vi "Home.vi"() -> ()   [LabVIEW 2015]
uses:
  <userlib>/QMH/Message Queue/Support/Enqueue Message (Single).vi
  <vilib>/Utility/error.llb/Error Cluster From Error Code.vi
  <vilib>/ErrorRing/Error Ring.xnode
  <userlib>/QMH/User Event - Stop/User Event - Stop.lvlib
  <userlib>/QMH/Message Queue/Message Queue.lvlib
panel:
  in  "Exit":bool
  in  "HostThread":variant
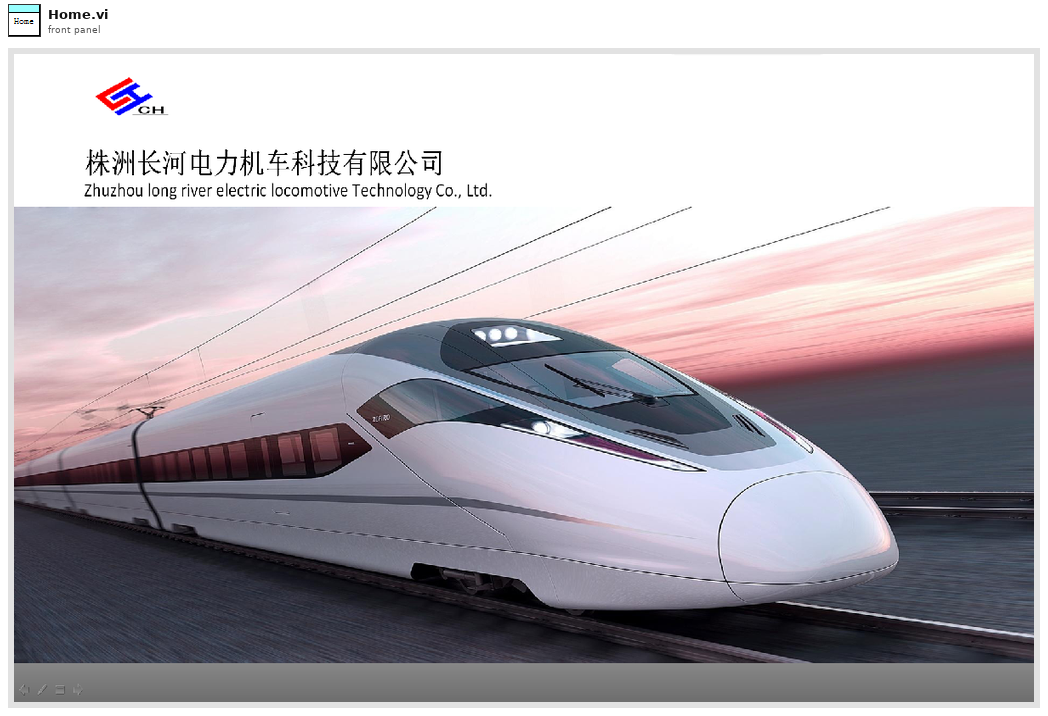
[diagram p1: front panel]
types:
  T1 = cluster{"Controls":cluster{"Exit":refnum<vi>}, "Thread":cluster{"ThisQ":string, "ThisVI":refnum<vi>, "HostQ":string, "HostRef":refnum<vi>, "SlavesQ":string[], "SlavesRef":refnum<vi>[]}, "Data":cluster{"Replace":bool}, "User":cluster{"Name":string}}
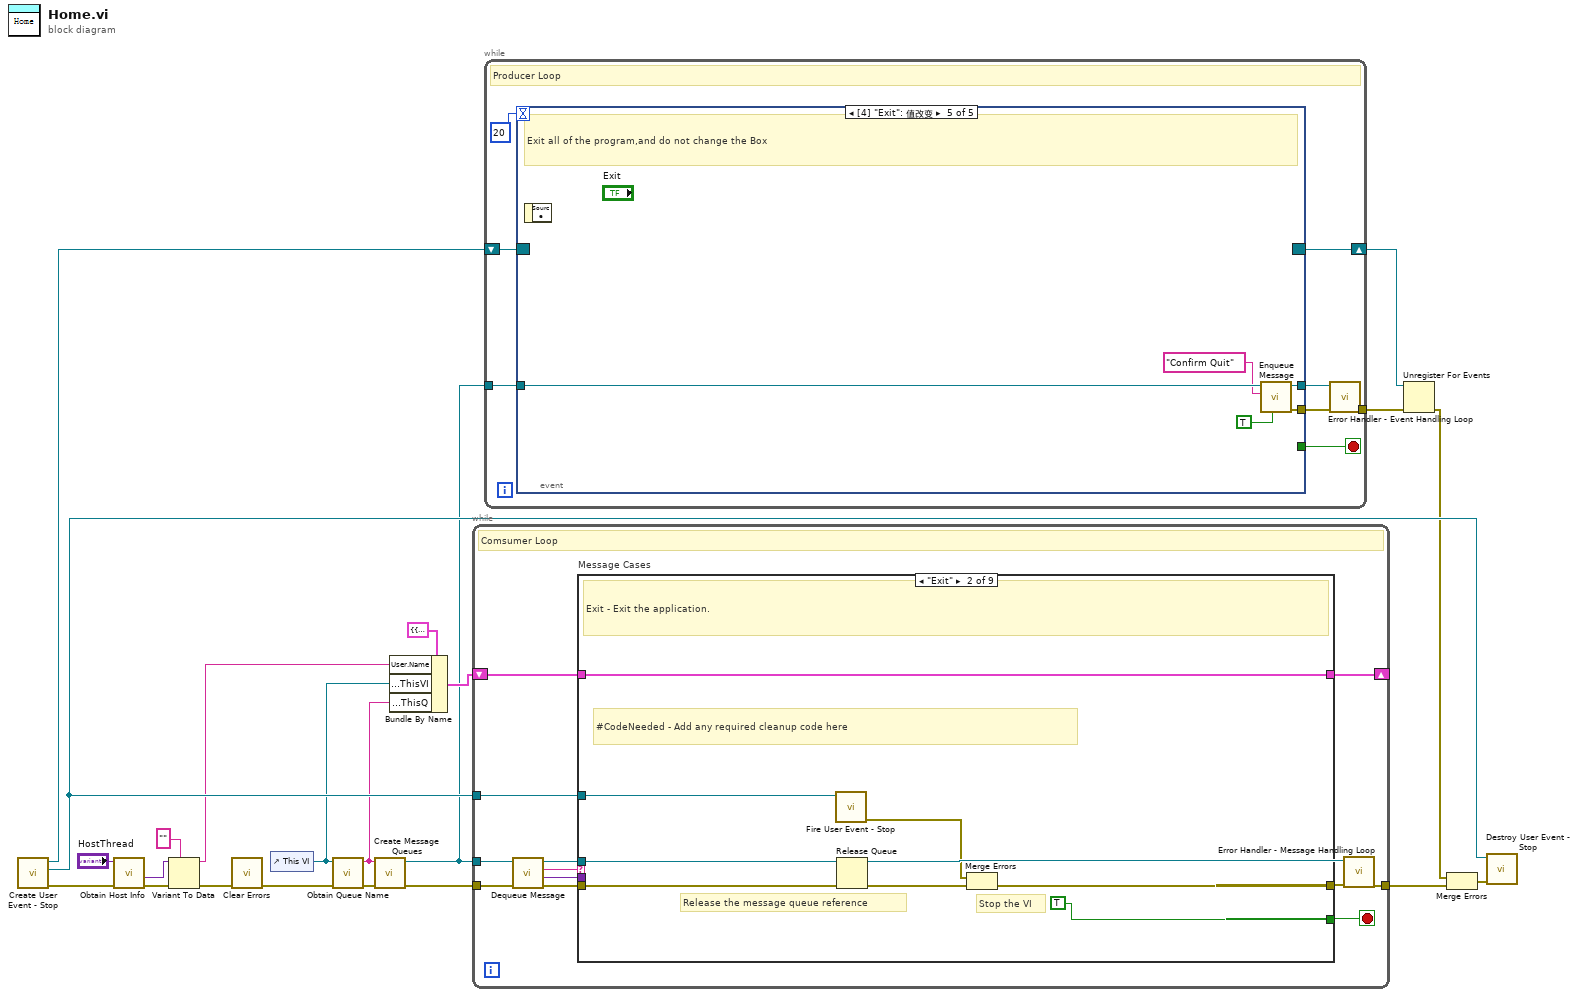
[diagram p0: block diagram]
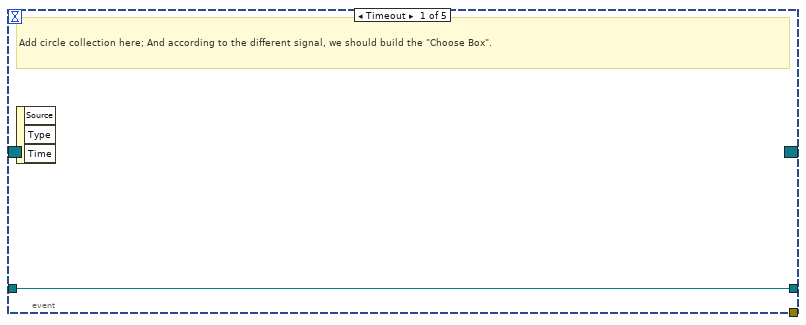
[diagram p2: hidden frame]
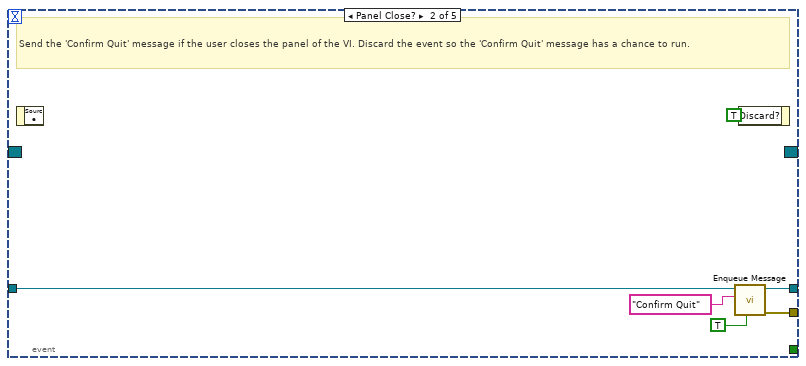
[diagram p3: hidden frame]
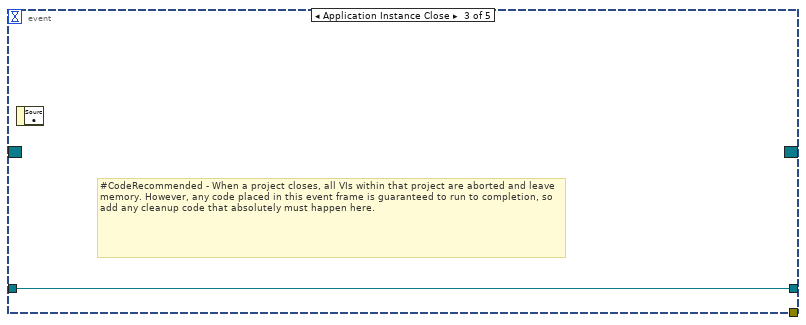
[diagram p4: hidden frame]
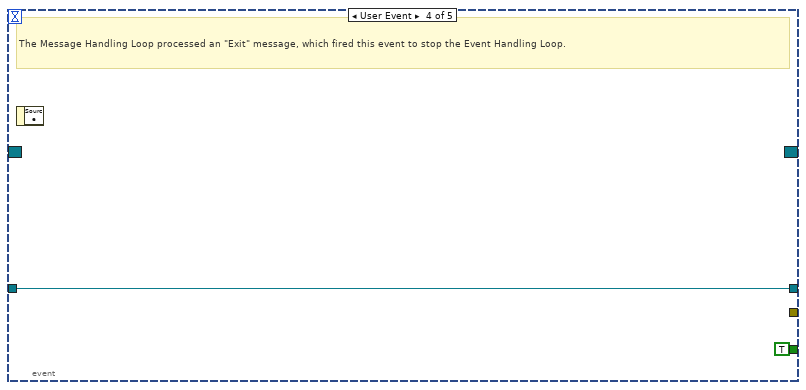
[diagram p5: hidden frame]
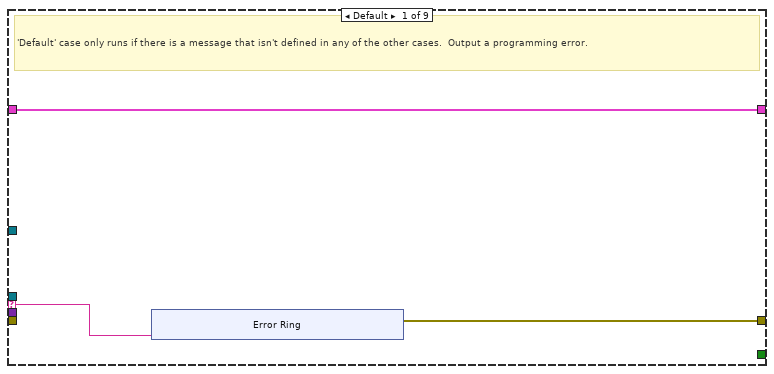
[diagram p6: hidden frame]
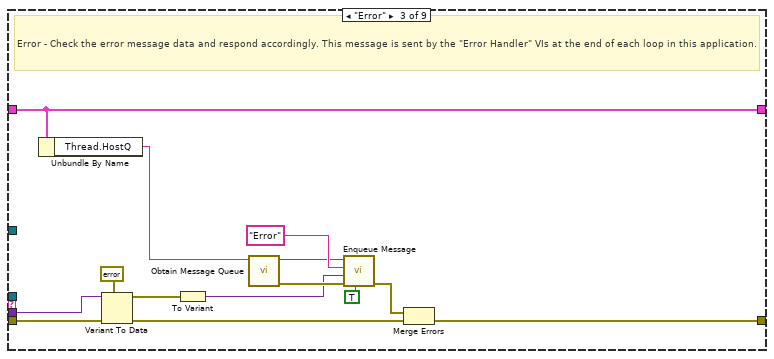
[diagram p7: hidden frame]
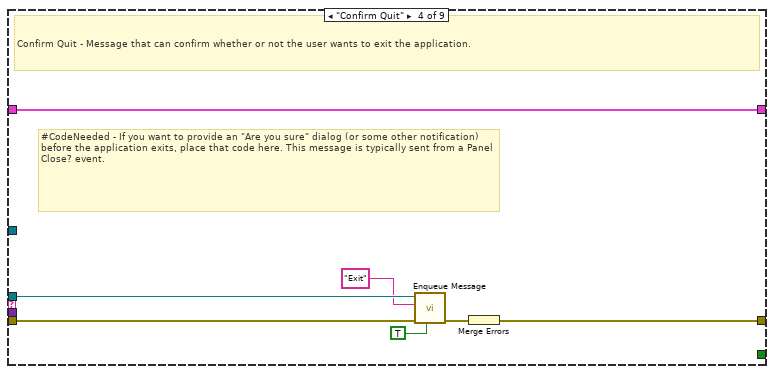
[diagram p8: hidden frame]
diagram:
  n1 = call <userlib>:"Create User Event - Stop.vi"() -> ("error out"=w9:errorcluster, "User Event - Stop"=w18:refnum<user-event>, "Stop Event Registration Refnum"=w20:refnum<event-registration>)  [unwired: 9 in]
  n2 = call <userlib>:"Obtain Host Info.vi"("error in (no error)"=w9, "HostThread"="HostThread") -> ("error out"=w6:errorcluster, "Data"=w5:variant)  [unwired: 6 in, 2 out]
  n3 = Variant To Data(error in=w6, type="", Variant=w5) -> (data=w1:string, error out=w3:errorcluster)
  n4 = call <vilib>:"Clear Errors.vi"("error in (no error)"=w3) -> ("error out"=w2:errorcluster)  [unwired: 5 in, 1 out]
  n5 = control-ref of="This VI"() -> (w11:refnum<vi>)
  n6 = call <userlib>:"Obtain Queue Name.vi"("error in (no error)"=w2, "VI Refnum"=w11) -> ("error out"=w14:errorcluster, "ViName"=w10:string)  [unwired: 8 in]
  n7 = call <userlib>:"Create Message Queues.vi"("error in (no error)"=w14, "name (unnamed)"=w10) -> ("error out"=w22:errorcluster, "QueueHandler"=w7:refnum<queue>)  [unwired: 8 in]
  n8 = Bundle By Name(cluster=T1 {"Controls"={"Exit"=refnum}, "Thread"={"ThisQ"="", "ThisVI"=refnum, "HostQ"="", "HostRef"=refnum, "SlavesQ"=[], "SlavesRef"=[]}, "Data"={"Replace"=FALSE}, "User"={"Name"=""}} ("Data Cluster"), "User.Name"=w1, "Thread.ThisVI"=w11, "Thread.ThisQ"=w10) -> (w12:T1)
  n9 = while {
    tunnel: w7 -> [w26]
    shift-right: [w33] -> _
    shift-left: w12 -> [w34]
    tunnel: w18 -> [w31]
    tunnel: w22 -> [w30]
    tunnel: [w24] -> w21
    stop <- w32 stop-if-true
    # "Comsumer Loop"
    n10 = call <userlib>:"Dequeue Message.vi"("error in (no error)"=w30, "Message Queue"=w26) -> ("error out"=w29:errorcluster, "Message Data"=w27:variant, "Message"=w28:string, "dup Message Queue"=w25:refnum<queue>)  [unwired: 6 in]
    n11 = case "Message Cases" shown="\"Exit\"" w28 {
      selector: w28 -> [w35 _ _ _ _ _ _ _ _]
      tunnel: w25 -> [_ w52 _ w69 _ _ _ _ _]
      tunnel: w29 -> [_ w47 w66 w73 w74 w77 w79 w80 w83]
      tunnel: [w36 w48 w61 w71 w74 w77 w79 w80 w83] -> w23
      tunnel: w34 -> [w37 w51 w58 w72 w75 w76 w78 w81 w82]
      tunnel: [w37 w51 w58 w72 w75 w76 w78 w81 w82] -> w33
      tunnel: [_ TRUE _ _ _ _ _ _ _] -> w32
      tunnel: w27 -> [_ _ w65 _ _ _ _ _ _]
      tunnel: w31 -> [_ w46 _ _ _ _ _ _ _]
      frame Default {
        # "'Default' case only runs if there is a message that isn't defined in any of the other cases.  Output a programming error."
        n12 = xnode "Error Ring"("参数 0"=w35) -> ("错误输出"=w36:errorcluster)
      }
      frame "Exit" {
        # "Stop the VI"
        # "Release the message queue reference"
        # "#CodeNeeded - Add any required cleanup code here"
        # "Exit - Exit the application."
        n13 = call <userlib>:"Fire User Event - Stop.vi"("User Event - Stop"=w46) -> ("error out"=w45:errorcluster)  [unwired: 10 in]
        n14 = Release Queue(queue=w52, error in (no error)=w47) -> (error out=w49:errorcluster)  [unwired: 1 in, 2 out]
        n15 = Merge Errors(w45, w49) -> (w48:errorcluster)
      }
      frame "Error" {
        # "Error - Check the error message data and respond accordingly. This message is sent by the \"Error Handler\" VIs at the end of each loop in this application."
        n16 = Unbundle By Name(w58) -> ("Thread.HostQ"=w57:string)
        n17 = Variant To Data(error in=w66, type=errorcluster {"status"=FALSE, "code"=0, "source"=""} ("error constant"), Variant=w65) -> (data=w54:errorcluster, error out=w63:errorcluster)
        n18 = To Variant(anything=w54) -> (Variant=w53:variant)
        n19 = call <userlib>:"Obtain Message Queue.vi"("name (unnamed)"=w57) -> ("error out"=w56:errorcluster, "Message Queue"=w55:refnum<queue>)  [unwired: 9 in]
        n20 = call-poly <userlib>:"Enqueue Message.vi"("Priority Message? (F)"=TRUE, "error in (no error)"=w56, "Message Data"=w53, "Message"="Error", "Message Queue"=w55) -> ("error out"=w62:errorcluster)  [unwired: 5 in, 1 out]
        n21 = Merge Errors(w62, w63) -> (w61:errorcluster)
      }
      frame "Confirm Quit" {
        # "#CodeNeeded - If you want to provide an \"Are you sure\" dialog (or some other notification) before the application exits, place that code here. This message is typically sent from a Panel Close? event."
        # "Confirm Quit - Message that can confirm whether or not the user wants to exit the application."
        n22 = call-poly <userlib>:"Enqueue Message.vi"("Priority Message? (F)"=TRUE, "error in (no error)"=w73, "Message"="Exit", "Message Queue"=w69) -> ("error out"=w70:errorcluster)  [unwired: 6 in, 1 out]
        n23 = Merge Errors(w70) -> (w71:errorcluster)
      }
      frame "Initialize" {
        # "Initialize - Send separate messages to initialize the data and the front panel.  Bundle control references."
      }
      frame "<-------UI-------->" {
      }
      frame "<------Core------>" {
      }
      frame "Core_InitializeRef" {
        # "Initialize control references. For there is not enough space to locate all the control references, separate the codes into 2 messages"
      }
      frame "<---Operation--->" {
      }
    }
    n24 = call <userlib>:"Error Handler - Message Handling Loop.vi"("error in (no error)"=w23, "Message Queue"=w25) -> ("dup error in"=w24:errorcluster)  [unwired: 8 in, 1 out]
  }
  n25 = while {
    tunnel: w7 -> [w91]
    shift-right: [w89] -> w16
    shift-left: w20 -> [w90]
    tunnel: [w85] -> w15
    stop <- w87 stop-if-true
    # "Producer Loop"
    n26 = event shown="[4] \"Exit\": 值改变" {
      selector: w90 -> [_ _ _ _ _]
      dyn-events: [_ _ _ _ _] -> w89
      timeout: 20 -> [_ _ _ _ _]
      tunnel: [_ _ _ TRUE ("Discard?") _] -> w87
      tunnel: w91 -> [w92 w97 w99 w101 w106]
      tunnel: [_ w96 _ _ w104] -> w88
      tunnel: [w92 w95 w99 w101 w105] -> w86
      event Timeout {
        # "Add circle collection here; And according to the different signal, we should build the \"Choose Box\"."
        n27 = event-data() -> ()  [unwired: 1 in, 3 out]
      }
      event Panel Close? {
        # "Send the 'Confirm Quit' message if the user closes the panel of the VI. Discard the event so the 'Confirm Quit' message has a chance to run."
        n28 = event-data() -> ()  [unwired: 1 in, 1 out]
        n29 = call-poly <userlib>:"Enqueue Message.vi"("Priority Message? (F)"=TRUE, "Message"="Confirm Quit", "Message Queue"=w97) -> ("error out"=w96:errorcluster, "dup Message Queue"=w95:refnum<queue>)  [unwired: 7 in]
        n30 = event-data("Discard?"=TRUE) -> ()  [unwired: 1 in, 1 out]
      }
      event Application Instance Close {
        # "#CodeRecommended - When a project closes, all VIs within that project are aborted and leave memory. However, any code placed in this event frame is guaranteed to run to completion, so add any cleanup code that absolutely must happen here."
        n31 = event-data() -> ()  [unwired: 1 in, 1 out]
      }
      event User Event {
        # "The Message Handling Loop processed an \"Exit\" message, which fired this event to stop the Event Handling Loop."
        n32 = event-data() -> ()  [unwired: 1 in, 1 out]
      }
      event "Exit": Value Change {
        # "Exit all of the program,and do not change the Box"
        n33 = event-data() -> ()  [unwired: 1 in, 1 out]
        n34 = call-poly <userlib>:"Enqueue Message.vi"("Priority Message? (F)"=TRUE, "Message"="Confirm Quit", "Message Queue"=w106) -> ("error out"=w104:errorcluster, "dup Message Queue"=w105:refnum<queue>)  [unwired: 7 in]
      }
    }
    n35 = call <userlib>:"Error Handler - Event Handling Loop.vi"("error in (no error)"=w88, "Message Queue"=w86) -> ("dup error in"=w85:errorcluster)  [unwired: 8 in, 1 out]
  }
  n36 = Unregister For Events(event registration refnum=w16, error in=w15) -> (error out=w17:errorcluster)
  n37 = Merge Errors(w17, w21) -> (w19:errorcluster)
  n38 = call <userlib>:"Destroy User Event - Stop.vi"("error in (no error)"=w19, "User Event - Stop"=w18) -> ()  [unwired: 9 in, 1 out]
